vi "getPositionsAndVoltages.vi"(0 "connection ID":refnum<k5>, 5 "error in":errorcluster) -> (14 "connection ID":refnum<k5>, 19 "error out":errorcluster)   [LabVIEW 2016]
doc: "Simultaneously get 3 axes positions as well as the DC offset\n to maximize sampling rate over network"
panel:
  out "val3":i32
  out "val2":i32
  out "val1":i32
  out "pos3":i32
  out "pos2":i32
  out "pos1":i32
  out "params_cluster":cluster{"Numeric":i32}
  in  "Params_cluster":cluster{"Numeric":dbl}
  in  "results_cluster":T1
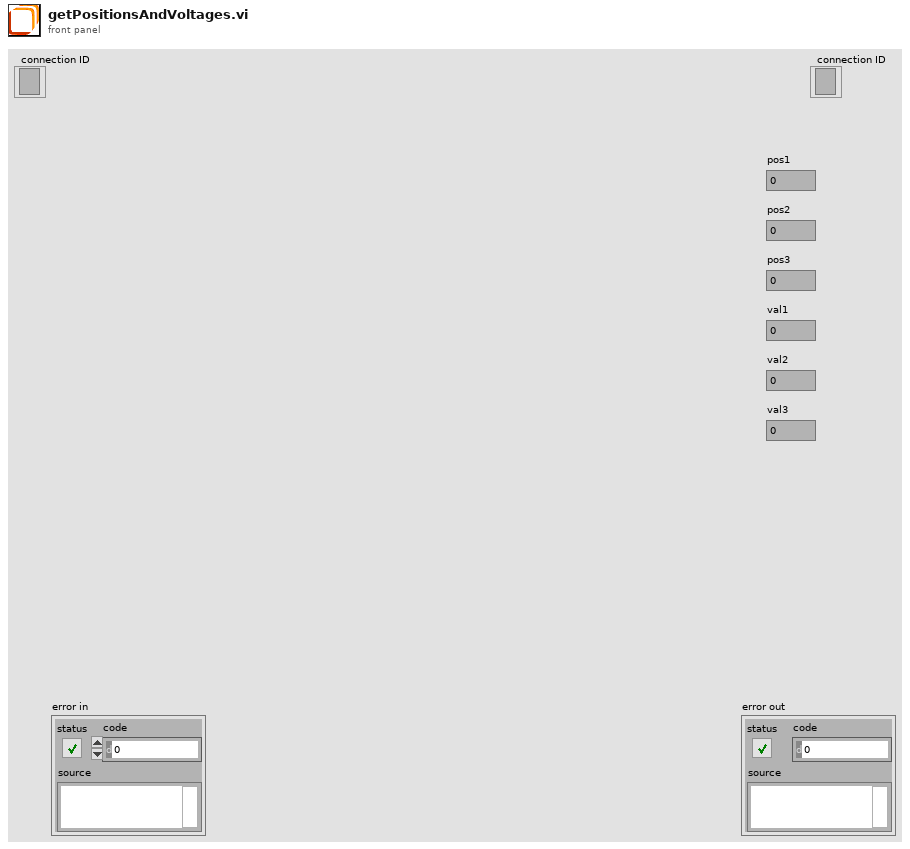
[diagram p1: front panel]
types:
  T1 = cluster{"errNo":i32, "pos1":i32, "pos2":i32, "pos3":i32, "val1":i32, "val2":i32, "val3":i32}
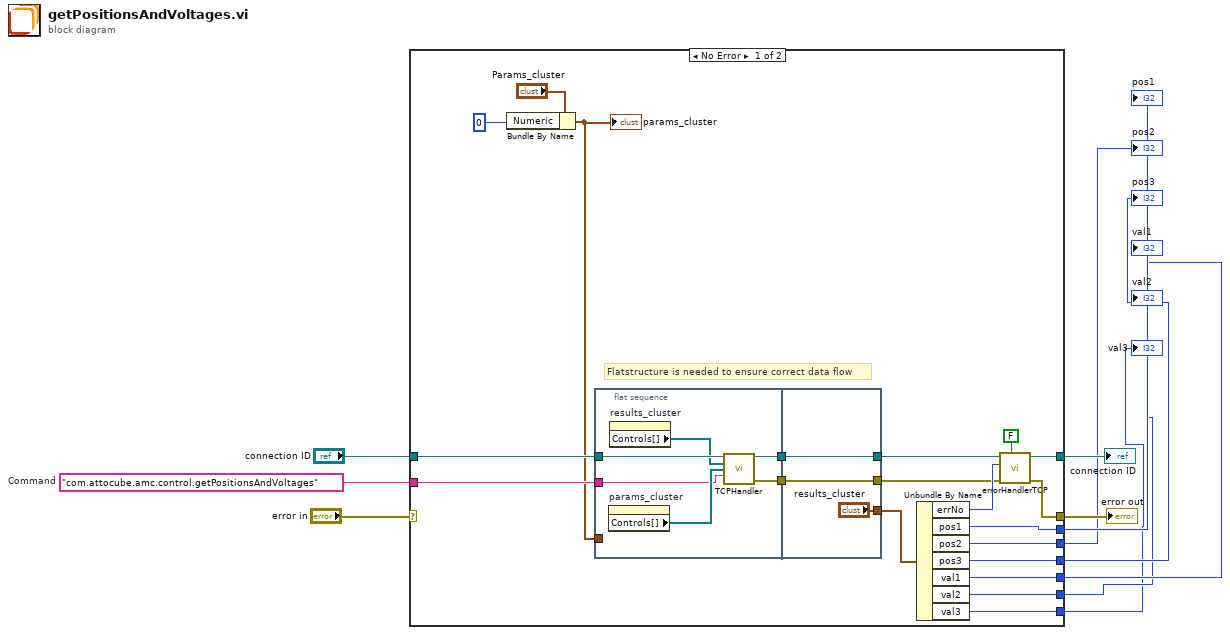
[diagram p0: block diagram]
diagram:
  w7 = "com.attocube.amc.control.getPositionsAndVoltages"  # Command
  n1 = case shown="No Error" "error in" {
    selector: "error in" -> [_ w42]
    tunnel: [w29 w42] -> w11
    tunnel: [w31 w41] -> w10
    tunnel: "connection ID" -> [w28 w41]
    tunnel: w7 -> [w22 _]
    tunnel: [w17 _] -> w6
    tunnel: [w16 _] -> w5
    tunnel: [w15 _] -> w4
    tunnel: [w14 _] -> w3
    tunnel: [w13 _] -> w2
    tunnel: [w12 _] -> w1
    frame No Error {
      # "Flatstructure is needed to ensure correct data flow"
      n2 = Bundle By Name(cluster="Params_cluster", "Numeric"=0) -> (w19:cluster{"Numeric":dbl})
      "params_cluster" <- w19
      n3 = flat-sequence {
        tunnel: [w36] -> w24
        tunnel: w28 -> [w37]
        tunnel: w22 -> [w33]
        tunnel: [w32] -> w20
        tunnel: w19 -> [_]
        tunnel: ["results_cluster"] -> w25
        tunnel: [w40] -> w27
        tunnel: w24 -> [w40]
        tunnel: [w38] -> w21
        tunnel: w20 -> [w38]
        frame #0 {
          n4 = property on="params_cluster" class="Clust (strict)"() -> ("Controls[]"=w34:refnum<vi>[])  [unwired: 2 in, 2 out]
          n5 = property on="results_cluster" class="Clust (strict)"() -> ("Controls[]"=w35:refnum<vi>[])  [unwired: 2 in, 2 out]
          n6 = call "TCPHandler.vi"("connection ID"=w37, "results_cluster"=w35, "params_cluster"=w34, "method"=w33) -> ("connection ID"=w36:refnum<k5>, "error"=w32:errorcluster)  [unwired: 8 in, 2 out]
        }
        frame #1 {
        }
      }
      n7 = Unbundle By Name(w25) -> ("errNo"=w26:i32, "pos1"=w17:i32, "pos2"=w16:i32, "pos3"=w15:i32, "val1"=w14:i32, "val2"=w13:i32, "val3"=w12:i32)
      n8 = call "errorHandlerTCP.vi"("show popup"=FALSE, "error in"=w21, "error number"=w26, "connection ID"=w27) -> ("error out"=w29:errorcluster, "connection ID"=w31:refnum<k5>)  [unwired: 6 in]
    }
    frame Error {
    }
  }
  "error out" <- w11
  "connection ID" <- w10
  "pos1" <- w6
  "pos2" <- w5
  "pos3" <- w4
  "val1" <- w3
  "val2" <- w2
  "val3" <- w1
